vi "IT-M7723 LIST Output.vi"() -> ()   [LabVIEW 2015]
doc: "This example is used to edit the parameters of the LIST, save them in the corresponding file, and run them."
uses:
  <instrlib>/IT-M7700/IT-M7700.lvlib
panel:
  in  "?":bool
  in  "Save File":u8=1 min=1 max=5
  in  "Jump To":u32=1 min=1 max=50 step=1
  in  "Repeat":u32=1 min=1 max=50000 step=1
  in  "End State":bool
  in  "Voltage Range":bool
  in  "LIST Parameter":T1(array[cluster]) {"Repeat" min=1 max=50000 step=1; "Kfreq" min=0.0; "Kdc" min=0.0; "Kac" min=0.0; "Stop Phase(°)" min=0.0 max=360.0; "Start Phase(°)" min=0.0 max=360.0; "Time(ms)" max=100000000; "Freq(Hz)" min=0.0; "Vdc(V)" min=0.0; "Vac(V)" min=0.0; "Level(%)" min=0.0 max=100.0; "Wave Type" max=39 step=1}
  in  "Serial Configuration":T2={"Baud Rate"=9600, "Parity"=0, "Data Bits"=8, "Stop Bits"=10, "Flow Control"=0} {"Flow Control" items=["None", "XON/XOFF", "RTS/CTS", "XON/XOFF & RTS/CTS", "DTR/DSR", "XON/XOFF & DTR/DSR"]; "Stop Bits" items=["1.0"=10, "1.5"=15, "2.0"=20]; "Data Bits" items=["7"=7, "8"=8]; "Parity" items=["None", "Odd", "Even", "Mark", "Space"]; "Baud Rate" items=["1200"=1200, "2400"=2400, "4800"=4800, "9600"=9600, "19200"=19200, "34800"=34800, "57600"=57600, "115200"=115200]}
  in  "VISA resource name":refnum<visa-resource-name>
  # "List Function"
  # "......"
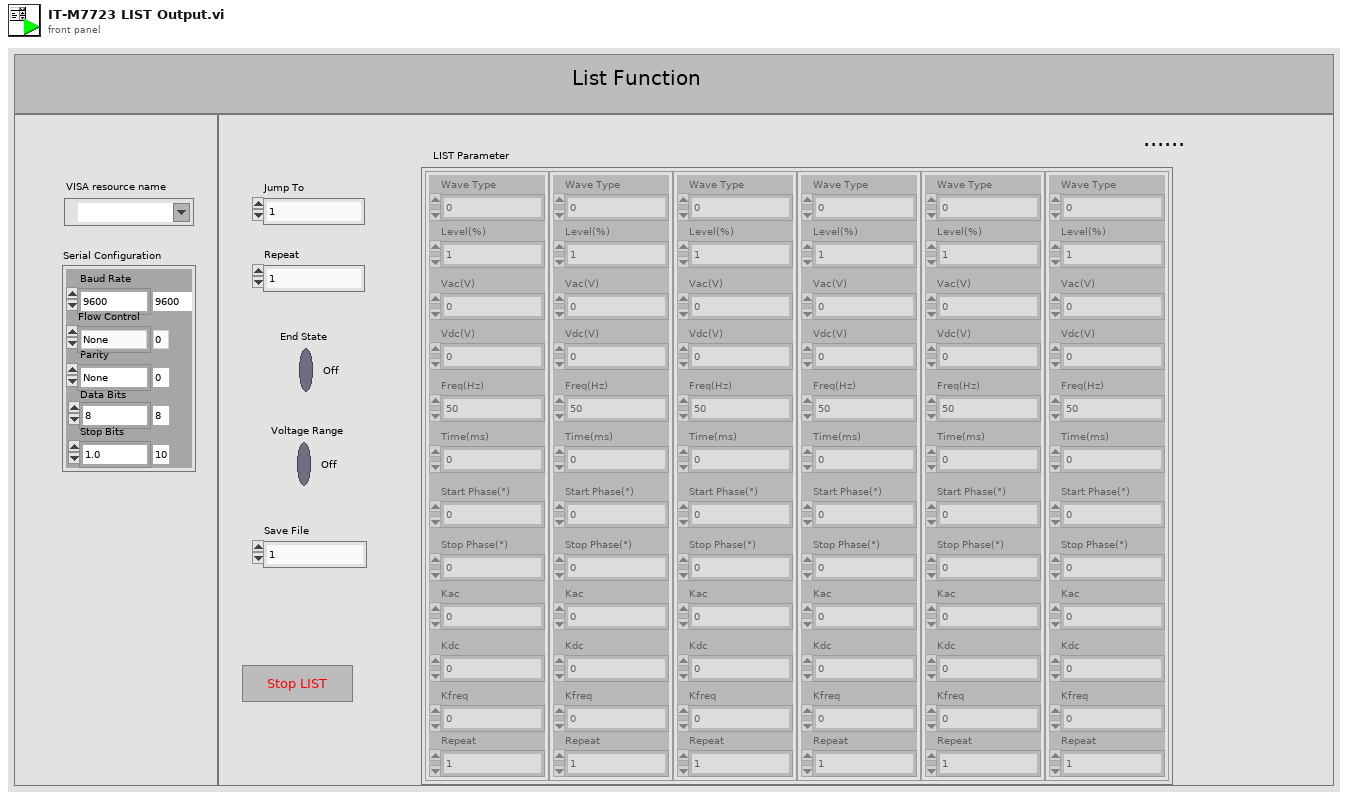
[diagram p1: front panel]
types:
  T1 = cluster{"Wave Type":u32, "Level(%)":dbl, "Vac(V)":dbl, "Vdc(V)":dbl, "Freq(Hz)":dbl, "Time(ms)":u32, "Start Phase(°)":dbl, "Stop Phase(°)":dbl, "Kac":dbl, "Kdc":dbl, "Kfreq":dbl, "Repeat":u32}[]
  T2 = cluster{"Baud Rate":u32, "Parity":u16, "Data Bits":u16, "Stop Bits":u16, "Flow Control":u16}
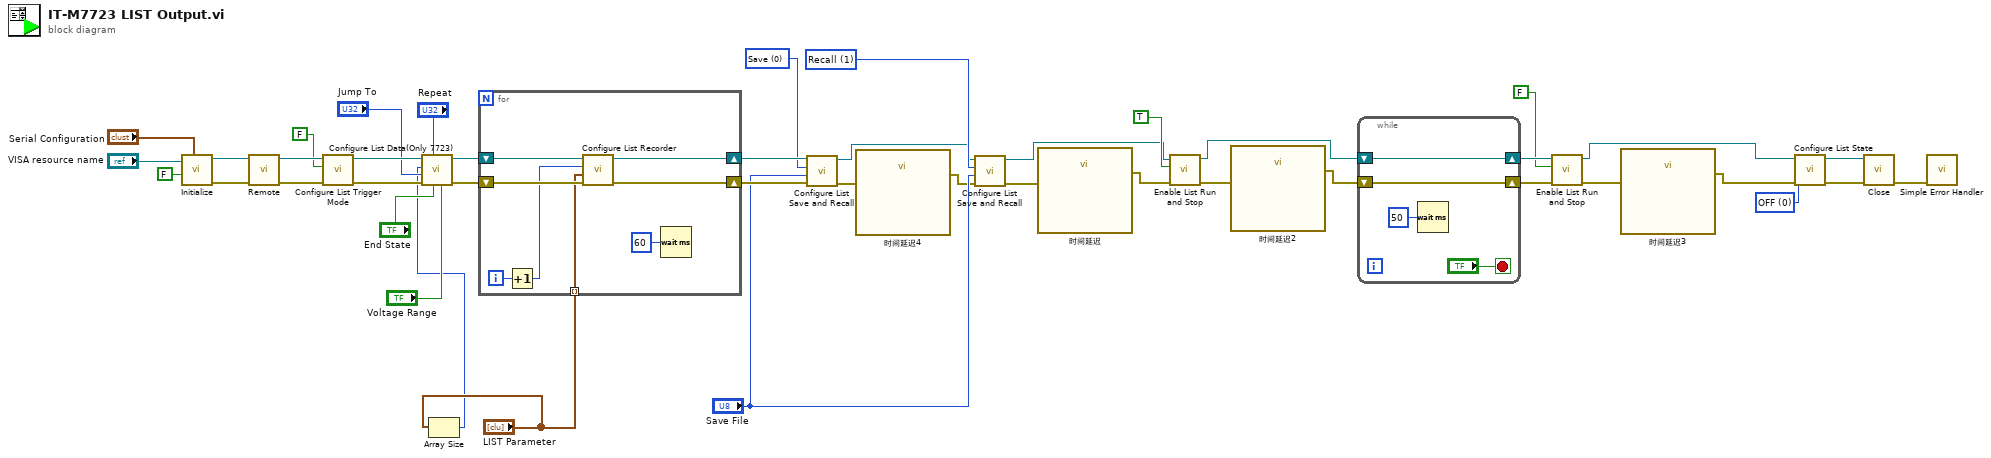
[diagram p0: block diagram]
diagram:
  w13 = u16 0 items=["OFF", " LIST1", " LIST2", " LIST3", " LIST4", " LIST5"] ("State")
  w24 = u16 1 items=["Save", "Recall"] ("Type")
  w25 = u16 0 items=["Save", "Recall"] ("Type")
  n1 = call <instrlib>:"Initialize.vi"("Serial Configuration"="Serial Configuration", "Reset"=FALSE, "VISA resource name"="VISA resource name") -> ("error out"=w40:errorcluster, "VISA resource name out"=w41:refnum<visa-resource-name>)  [unwired: 7 in]
  n2 = call <instrlib>:"Remote.vi"("error in"=w40, "VISA resource name"=w41) -> ("error out"=w37:errorcluster, "VISA resource name out"=w38:refnum<visa-resource-name>)  [unwired: 8 in]
  n3 = call <instrlib>:"Configure List Trigger Mode.vi"("error in"=w37, "Mode"=FALSE, "VISA resource name"=w38) -> ("error out"=w35:errorcluster, "VISA resource name out"=w34:refnum<visa-resource-name>)  [unwired: 7 in]
  n4 = Array Size(array="LIST Parameter") -> (size(s)=w18:i32)
  n5 = call <instrlib>:"Configure List Data(Only 7723).vi"("Range"="Voltage Range", "End State"="End State", "Repeat"="Repeat", "error in"=w35, "Jump To"="Jump To", "Record Num"=w18, "VISA resource name"=w34) -> ("error out"=w33:errorcluster, "VISA resource name out"=w32:refnum<visa-resource-name>)  [unwired: 3 in]
  n6 = for {
    shift-right: [w49] -> w27
    shift-left: w32 -> [w51]
    shift-right: [w48] -> w26
    shift-left: w33 -> [w50]
    tunnel: "LIST Parameter" -> [w45] mode=indexing
    i -> [w47]
    n7 = Increment(x=w47) -> (x+1=w46:i32)
    n8 = call <instrlib>:"Configure List Recorder.vi"("error in"=w50, "Parameter"=w45, "Step"=w46, "VISA resource name"=w51) -> ("error out"=w48:errorcluster, "VISA resource name out"=w49:refnum<visa-resource-name>)  [unwired: 6 in]
    n9 = Wait (ms)(milliseconds to wait=u32 60 ("等待时间（毫秒）")) -> ()  [unwired: 1 out]
  }
  n10 = call <instrlib>:"Configure List Save and Recall.vi"("error in"=w26, "File"="Save File", "Type"=w25, "VISA resource name"=w27) -> ("error out"=w9:errorcluster, "VISA resource name out"=w10:refnum<visa-resource-name>)  [unwired: 6 in]
  n11 = call "时间延迟4"("error in (no error)"=w9) -> ("error out"=w8:errorcluster)  [unwired: 10 in]
  n12 = call <instrlib>:"Configure List Save and Recall.vi"("error in"=w8, "File"="Save File", "Type"=w24, "VISA resource name"=w10) -> ("error out"=w6:errorcluster, "VISA resource name out"=w7:refnum<visa-resource-name>)  [unwired: 6 in]
  n13 = call "时间延迟"("error in (no error)"=w6) -> ("error out"=w5:errorcluster)  [unwired: 10 in]
  n14 = call <instrlib>:"Enable List Run and Stop.vi"("error in"=w5, "State"=TRUE, "VISA resource name"=w7) -> ("error out"=w15:errorcluster, "VISA resource name out"=w16:refnum<visa-resource-name>)  [unwired: 7 in]
  n15 = call "时间延迟2"("error in (no error)"=w15) -> ("error out"=w14:errorcluster)  [unwired: 10 in]
  n16 = while {
    shift-right: [w55] -> w21
    shift-left: w16 -> [w55]
    shift-right: [w54] -> w20
    shift-left: w14 -> [w54]
    stop <- "?" stop-if-true
    n17 = Wait (ms)(milliseconds to wait=u32 50 ("等待时间（毫秒）")) -> ()  [unwired: 1 out]
  }
  n18 = call <instrlib>:"Enable List Run and Stop.vi"("error in"=w20, "State"=FALSE, "VISA resource name"=w21) -> ("error out"=w3:errorcluster, "VISA resource name out"=w4:refnum<visa-resource-name>)  [unwired: 7 in]
  n19 = call "时间延迟3"("error in (no error)"=w3) -> ("error out"=w2:errorcluster)  [unwired: 10 in]
  n20 = call <instrlib>:"Configure List State.vi"("error in"=w2, "State"=w13, "VISA resource name"=w4) -> ("error out"=w11:errorcluster, "VISA resource name out"=w12:refnum<visa-resource-name>)  [unwired: 7 in]
  n21 = call <instrlib>:"Close.vi"("error in"=w11, "VISA resource name"=w12) -> ("error out"=w39:errorcluster)  [unwired: 9 in]
  n22 = call <vilib>:"Simple Error Handler.vi"("error in (no error)"=w39) -> ()  [unwired: 4 in, 5 out]
